vi "CreateSerializationSession.vi"(8 "error in (no error)":errorcluster) -> (0 "error out":errorcluster, 3 "Serialization Session ID":T1)   [LabVIEW 2019, in "Template Client.lvlib" / "gprc-lvsupport.lvlib"]
uses:
  gprc-lvsupport.lvlib
  typeDefs/grpcId.ctl
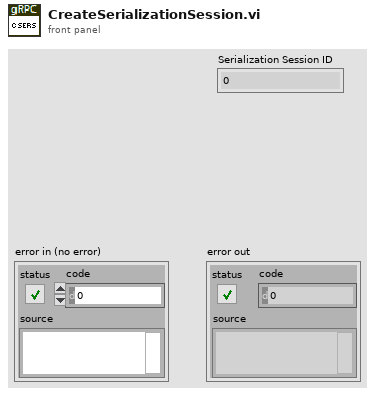
[diagram p1: front panel]
types:
  T1 = typedef "Template Client.lvlib/gprc-lvsupport.lvlib/grpcId.ctl" = u64
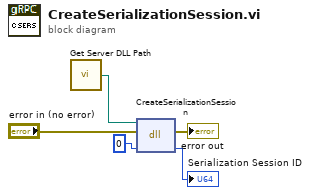
[diagram p0: block diagram]
diagram:
  n1 = call "Get Server DLL Path.vi"() -> ("Server dll path"=w4:path)
  n2 = dll-call lib="?" fn="CreateSerializationSession"(path in=w4, error in="error in (no error)", "serializationId"=u64 0 ("gRPCId")) -> (error out=→"error out":errorcluster, "serializationId"=→"Serialization Session ID":u64)  [unwired: 2 in, 1 out]
